vi "write-csv_file.vi"() -> ()   [LabVIEW 2024]
uses:
  <vilib>/Utility/file.llb/Write Delimited Spreadsheet (string).vi
panel:
  in  "Cluster":T1 {"Edad" format="%#_13g"}
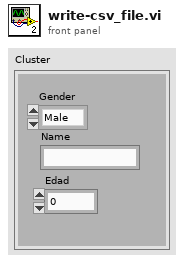
[diagram p1: front panel]
types:
  T1 = cluster{"Gender":enum16{"Male", "Female"}, "Name":string, "Edad":dbl}
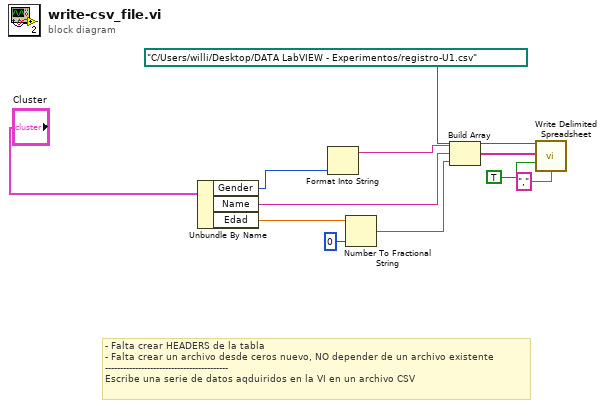
[diagram p0: block diagram]
diagram:
  # "- Falta crear HEADERS de la tabla\n- Falta crear un archivo desde ceros nuevo, NO depender de un archivo existente\n-----------------------------------------\nEscribe una serie de datos aqduiridos en la VI en un archivo CSV"
  n1 = Unbundle By Name("Cluster") -> ("Gender"=w8:enum16{"Male", "Female"}, "Name"=w6:string, "Edad"=w10:dbl)
  n2 = Format Into String(w8) -> (resulting string=w7:string)  [unwired: 3 in, 1 out]
  n3 = Number To Fractional String(number=w10, precision (6)=i16 0) -> (F-format string=w5:string)  [unwired: 2 in]
  n4 = Build Array(w7, w6, w5) -> (w4:string[])
  n5 = call-poly <vilib>:"Write Delimited Spreadsheet.vi"("file path (dialog if empty)"=path "C:/Users/willi/Desktop/DATA LabVIEW - Experimentos/registro-U1.csv", "1D data"=w4, "append to file? (new file:F)"=TRUE, "delimiter (\\t)"="," ("delimiter (\\t)")) -> ()  [unwired: 10 in, 2 out]
